vi "LS_372_still_control.vi"(4 "Still Resistance":dbl, 5 "Still Power":dbl, 6 "Still heater":bool, 7 "VISA-Ressourcenname":refnum<visa-resource-name>) -> ()   [LabVIEW 2018]
uses:
  Equipment/Lake Shore 372/Lake Shore 372.lvlib
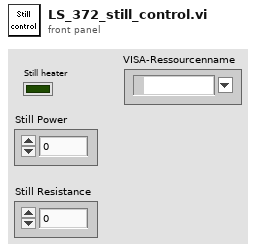
[diagram p1: front panel]
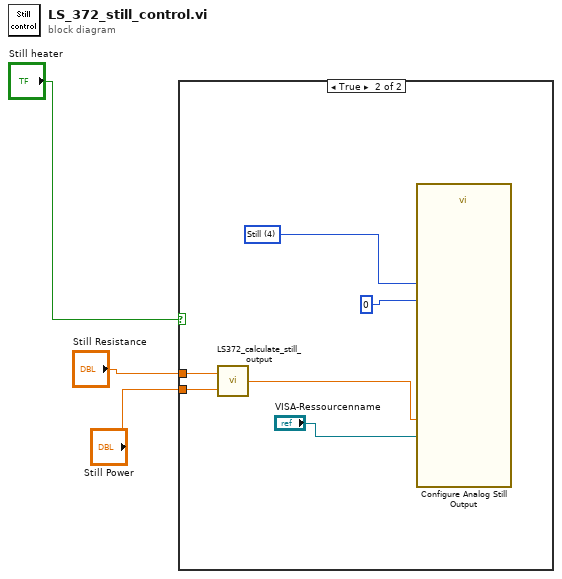
[diagram p0: block diagram]
diagram:
  n1 = case shown="True" "Still heater" {
    tunnel: "Still Power" -> [_ w7]
    tunnel: "Still Resistance" -> [_ w6]
    frame False {
    }
    frame True {
      w9 = u16 4 items=["Off"=0, "Monitor Out"=1, "Open Loop (Manual)"=2, "Still"=4] ("Analog Out Mode (0: Off)")
      n2 = call "LS372_calculate_still_output.vi"("Power (mW)"=w7, "Resistance (Ohms)"=w6) -> ("Analog Output (%)"=w4:dbl)
      n3 = call "Configure Analog Still Output.vi"("VISA resource name"="VISA-Ressourcenname", "Analog Out Mode (0: Off)"=w9, "Channel (1:1)"=0, "Still Value (0.000%)"=w4) -> ()  [unwired: 10 in, 2 out]
    }
  }
